vi "StopScan.vi"(0 "Close FP":bool, 1 "Motion Settings In":T5={"No Motion?"=FALSE, "Motion System"=enum."NI 735x", "Motion Bd ID"=1, "Motion Profile"="SMAC1", "# Axis"=1, "Reverse Z axis?"=TRUE, "SMAC Axis"=0, "scan pair"=enum."y-(x) scan", "RT fps"=6.0, "Steps per mm"=[1000, 1000, 1000, 1000], "Motor Parameters"={"velocity ct/s"=[10000.0, 10000.0, 10000.0, 50000.0], "accel ct/s^2"=[50000.0, 50000.0, 50000.0, 200000.0]}, "One Way Scan"=FALSE, "Reverse One Way Scan"=FALSE, "Global Position (mm)"=[], "Plane"=0, "Distance between\nscan lines (um)"=0.0, "Distance between\nscan planes (um)"=0.0, "number of scan planes"=1, "Total steps in line"=0, "Xtra plane\ndistance  (um)"=100, "Xtra planes "=1, "Add Axis"=FALSE, "overshoot cts"=200, "BKPT Shift"=0, "Scan Start Time (ms)"=0, "ESP VISA"="GPIB::1::INSTR", "3rd Axis"=1, "GL Ref Out"=refnum, "Galil Address"=""} {"3rd Axis" items=["x", "y", "z", "w"]; "Xtra planes" min=1; "Xtra plane\ndistance  (um)" min=0; "Distance between\nscan planes (um)" format="%.2f"; "Distance between\nscan lines (um)" format="%.2f"; "SMAC Axis" items=["None"=0, "Axis 1"=1, "Axis 2"=2, "Axis 3"=3, "Axis 4"=4, "Axis 5"=5, "Axis 6"=6, "Axis 7"=7, "Axis 8"=8, "Vector Space 1"=17, "Vector Space 2"=18, "Vector Space 3"=19, "Vector Space 4"=20]; "Motion Bd ID" min=1 max=32 step=1}, 2 "Ring":i32, 4 "Digitizer Settings":T1={"Digitizer delay (us) "=0.0, "rf points per line"=2048, "lines per plane"=128, "Samp Rate (Hz)"=100000000.0, "Additional dig delay (us)"=0.0, "Voltage Scale"=0.4, "Pre-Looks"=0, "Offset delay (us)"=0.0, "bits A/D"=8, "Avg Num"=1, "DigTimeOut"=5.0, "Rel Dig Delay"=0.0, "Dig Ch"=0, "LeCroyCluster"={"LeCroy Channels"=[TRUE, FALSE, FALSE, FALSE], "LC read pt offset"=0.0, "Sweep Avg"=FALSE}, "Main Digitizer"=enum."NI Digitizer", "Dig Config"=enum."Single channel", "Digitizer ID Cluster"={"Acqiris/Alazar/SP ID"=[], "NI Instr Handles"=[], "LeCroy VISA"="", "GaGe Handle"={"Handle"=0, "Sample size"=0, "Resolution"=0, "Offset"=0, "Channels"=0, "Boards"=0}, "ATS Ref"="ATS9350", "Acqiris Address"=["PCI::INSTR0"], "ADQRef"=refnum, "adq_cu_ptr"=refnum}, "Trigger Settings"={"Trig Source"=1, "Trig Coupling"=0, "Trig Slope"=0, "Level (mV)"=1500.0}, "Bulk Acq"=FALSE, "Bulk Start Indexes"=[], "Data Ref RF"=refnum, "NI ID/Channel"=[], "Total Dig CH"=1, "Xtra Ann Trig delay (us)"=10.0, "Fix Z Delay?"=FALSE, "One Way Transmission?"=FALSE, "Data Ref Log"=refnum} {"Trigger Settings"."Trig Slope" items=["Positive", "Negative"]; "Trigger Settings"."Level (mV)" format="%.2f"; "Trigger Settings"."Trig Coupling" items=["DC 1 MOhm", "AC 1 MOhm", "DC 50 Ohm", "AC 50 Ohm"]; "Trigger Settings"."Trig Source" items=["Chan 1", "External"]; "Rel Dig Delay" format="%.2f"; "DigTimeOut" format="%.2f"; "Avg Num" min=1; "Offset delay (us)" format="%.2f"; "Additional dig delay (us)" format="%.2f"; "Digitizer delay (us)" format="%.2f"}, 6 "Line Number":i32) -> (5 "Stop Now? Dup":bool)   [LabVIEW 2022 SP3]
uses:
  Motion Controllers/NI_controller/-NI_MotionRoutines/MotionParameters.ctl
  Motion Controllers/NI_controller/-NI_MotionRoutines/MotionSys.ctl
  Motion Controllers/-MotionRoutines/ScanAxis.ctl
  Motion Controllers/-MotionRoutines/3rdAxis.ctl
  Digitizers/-DigitizerRoutines/DigitizerSettings.ctl
  Digitizers/-DigitizerRoutines/Digitizer.ctl
  Digitizers/-DigitizerRoutines/DigConfig.ctl
  Digitizers/-DigitizerRoutines/DigitizerID.ctl
  C:/Windows/System32/ADQAPI_dotNet_helper.dll
panel:
  in  "Alert when done?":bool=TRUE
  out "Minutes Remaining":dbl format="%.1f"
  out "Progress":u8(slide) scale=0.0..100.0
  in  "Pause?":bool
  in  "Current Plane":i32
  in  "Stop Now?":bool
  # "Can pause or stop mid-scan"
  # "1-D and 2-D B scan settings"
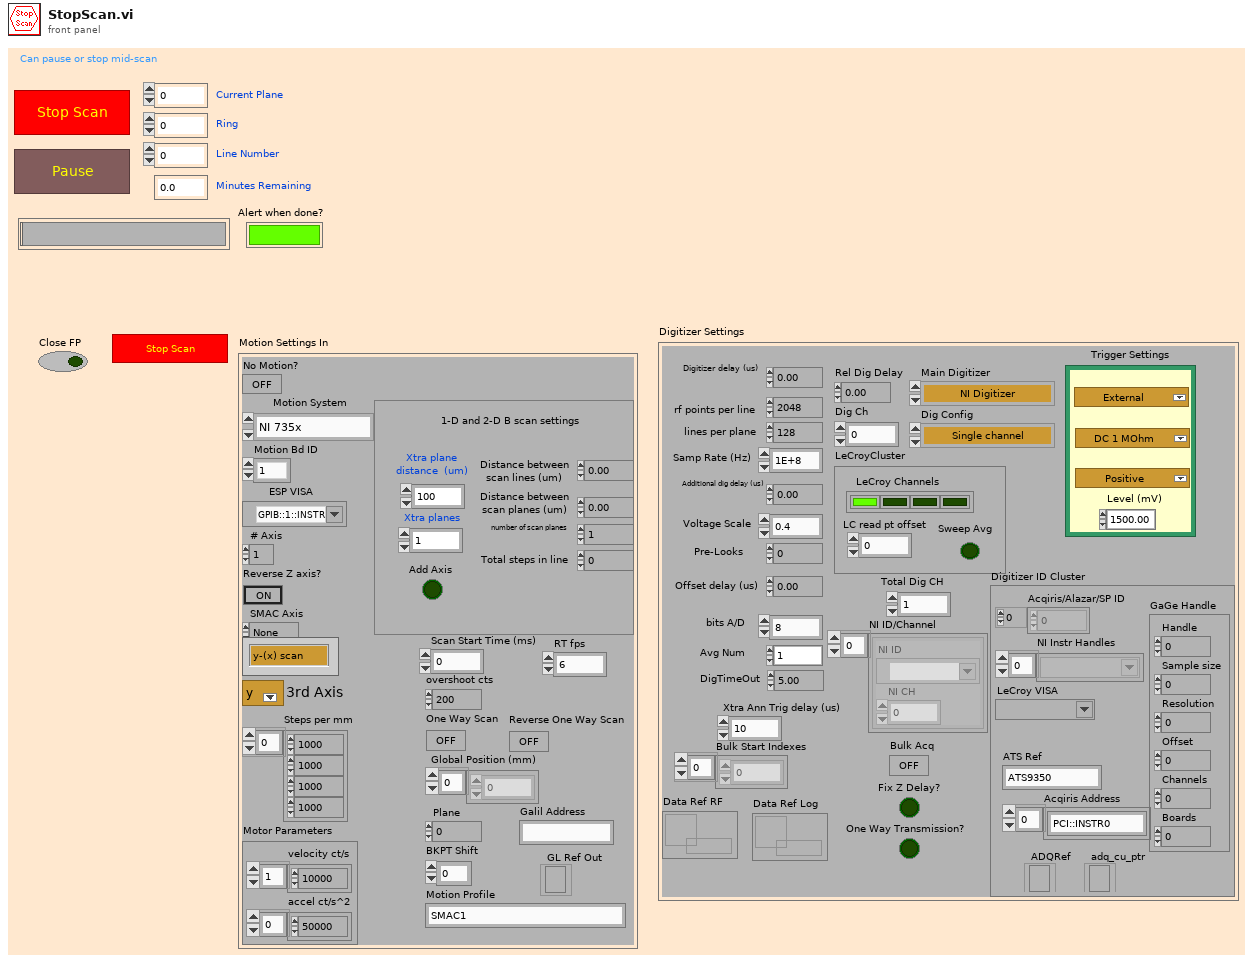
[diagram p1: front panel]
types:
  T1 = typedef "DigitizerSettings.ctl" = cluster{"Digitizer delay (us) ":dbl, "rf points per line":i32, "lines per plane":i32, "Samp Rate (Hz)":dbl, "Additional dig delay (us)":dbl, "Voltage Scale":dbl, "Pre-Looks":i32, "Offset delay (us)":dbl, "bits A/D":i8, "Avg Num":i32, "DigTimeOut":sgl, "Rel Dig Delay":sgl, "Dig Ch":i32, "LeCroyCluster":cluster{"LeCroy Channels":bool[], "LC read pt offset":dbl, "Sweep Avg":bool}, "Main Digitizer":T2, "Dig Config":T3, "Digitizer ID Cluster":T4, "Trigger Settings":cluster{"Trig Source":u16, "Trig Coupling":u16, "Trig Slope":u16, "Level (mV)":dbl}, "Bulk Acq":bool, "Bulk Start Indexes":i32[], "Data Ref RF":refnum<data-value>, "NI ID/Channel":cluster{"NI ID":refnum<k15>, "NI CH":i32}[], "Total Dig CH":i32, "Xtra Ann Trig delay (us)":dbl, "Fix Z Delay?":bool, "One Way Transmission?":bool, "Data Ref Log":refnum<data-value>}
  T2 = typedef "Digitizer.ctl" = enum16{"Acqiris Digitizer", "NI Digitizer", "LeCroy", "GaGe", "AlazarTech", "No Digitizer", "Teledyne"}
  T3 = typedef "DigConfig.ctl" = enum16{"Single channel", "2 Chans w/ 2 Acqiris", "2 Chans w/ 1 Acqiris", "5-CH Pulser New", "5-CH pulser w/ ann array", "5-pass style ann array", "Empty"}
  T4 = typedef "DigitizerID.ctl" = cluster{"Acqiris/Alazar/SP ID":u32[], "NI Instr Handles":refnum<k15>[], "LeCroy VISA":refnum<visa-resource-name>, "GaGe Handle":cluster{"Handle":u32, "Sample size":u32, "Resolution":i32, "Offset":i32, "Channels":u32, "Boards":u32}, "ATS Ref":string, "Acqiris Address":string[], "ADQRef":refnum<k24>, "adq_cu_ptr":refnum<k24>}
  T5 = typedef "MotionParameters.ctl" = cluster{"No Motion?":bool, "Motion System":T6, "Motion Bd ID":u8, "Motion Profile":string, "# Axis":i8, "Reverse Z axis?":bool, "SMAC Axis":u16, "scan pair":T7, "RT fps":sgl, "Steps per mm":i32[], "Motor Parameters":cluster{"velocity ct/s":dbl[], "accel ct/s^2":dbl[]}, "One Way Scan":bool, "Reverse One Way Scan":bool, "Global Position (mm)":dbl[], "Plane":i32, "Distance between\nscan lines (um)":sgl, "Distance between\nscan planes (um)":sgl, "number of scan planes":i32, "Total steps in line":i32, "Xtra plane\ndistance  (um)":i32, "Xtra planes ":i32, "Add Axis":bool, "overshoot cts":i32, "BKPT Shift":i32, "Scan Start Time (ms)":u32, "ESP VISA":refnum<visa-resource-name>, "3rd Axis":T8, "GL Ref Out":refnum<k7>, "Galil Address":string}
  T6 = typedef "MotionSys.ctl" = enum16{"MM3000", "NI 735x", "Newport ESP", "No Motion Card", "Galil"}
  T7 = typedef "ScanAxis.ctl" = enum16{"y-(x) scan", "x-(y) scan", "z-(x) scan", "z-(y) scan", "y-(z) scan", "x-(z) scan", "w-(x) scan", "w-(y) scan", "w-(z) scan", "x-(w) scan", "y-(w) scan", "z-(w) scan"}
  T8 = typedef "3rdAxis.ctl" = u16
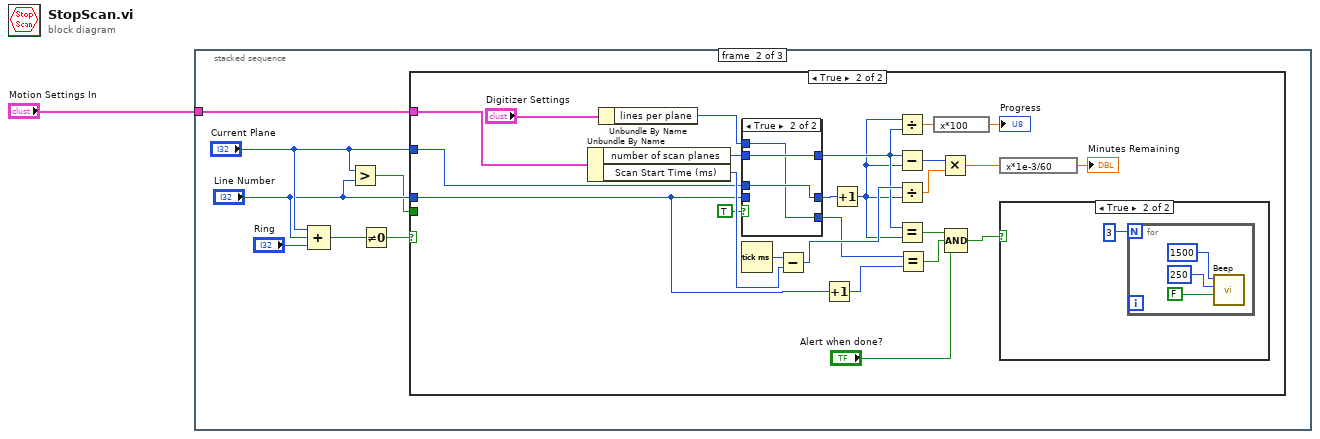
[diagram p0: block diagram]
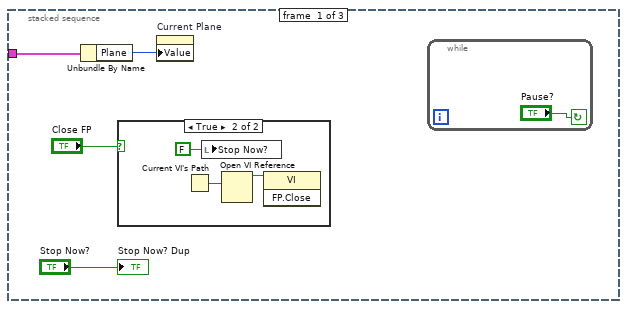
[diagram p2: hidden frame]
diagram:
  n1 = stacked-sequence {
    tunnel: "Motion Settings In" -> [w2 w10 _]
    frame #0 {
      n2 = Unbundle By Name(w2) -> ("Plane"=w3:i32)
      n3 = case shown="True" "Close FP" {
        frame False {
        }
        frame True {
          n4 = Current VI's Path() -> (path=w9:path)
          n5 = local write "Stop Now?"(FALSE) -> ()
          n6 = Open VI Reference(vi path=w9) -> (vi reference=w8:refnum<vi>)  [unwired: 2 in, 4 out]
          n7 = invoke class="VI" method="FP.Close"(reference=w8) -> ()  [unwired: 2 in, 3 out]
        }
      }
      n8 = property on="Current Plane" class="DigNum (strict)"("Value"=w3) -> ()  [unwired: 2 in, 2 out]
      n9 = while {
        stop <- "Pause?" continue-if-true
      }
      "Stop Now? Dup" <- "Stop Now?"
    }
    frame #1 {
      n10 = Compound Arithmetic op=ADD("Current Plane", "Line Number", "Ring") -> (w16:i32)
      n11 = Greater?(x="Current Plane", y="Line Number") -> (0:w11:bool)
      n12 = Not Equal To 0?(x=w16) -> (x != 0?=w15:bool)
      n13 = case shown="True" w15 {
        tunnel: "Current Plane" -> [_ w28]
        tunnel: w11 -> [_ _]
        tunnel: "Line Number" -> [_ w18]
        tunnel: w10 -> [_ w24]
        frame False {
        }
        frame True {
          n14 = Unbundle By Name(w24) -> ("number of scan planes"=w26:i32, "Scan Start Time (ms)"=w33:u32)
          n15 = Unbundle By Name("Digitizer Settings") -> ("lines per plane"=w25:i32)
          n16 = case shown="True" TRUE {
            tunnel: [w43 w46] -> w29
            tunnel: w28 -> [_ w46]
            tunnel: w18 -> [w43 _]
            tunnel: [w42 w45] -> w27
            tunnel: w26 -> [_ w45]
            tunnel: w25 -> [w42 w44]
            tunnel: [w42 w44] -> w22
            frame False {
            }
            frame True {
            }
          }
          n17 = Tick Count (ms)() -> (millisecond timer value=w41:u32)
          n18 = Subtract(x=w41, y=w33) -> (x-y=w34:u32)
          n19 = Increment(x=w18) -> (x+1=w17:i32)
          n20 = Increment(x=w29) -> (x+1=w21:i32)
          n21 = Divide(x=w21, y=w27) -> (x/y=w40:dbl)
          n22 = Subtract(x=w27, y=w21) -> (x-y=w39:i32)
          n23 = Divide(x=w34, y=w21) -> (x/y=w38:dbl)
          n24 = Equal?(x=w27, y=w21) -> (x = y?=w31:bool)
          n25 = Equal?(x=w22, y=w17) -> (x = y?=w20:bool)
          n26 = expression code="x*100"(w40) -> (→"Progress":dbl)
          n27 = Multiply(x=w39, y=w38) -> (x*y=w37:dbl)
          n28 = Compound Arithmetic op=AND(w31, w20, "Alert when done?") -> (w32:bool)
          n29 = expression code="x*1e-3/60"(w37) -> (→"Minutes Remaining":dbl)
          n30 = case shown="True" w32 {
            frame False {
            }
            frame True {
              n31 = for {
                N: 3 -> [_]
                n32 = call <vilib>:"Beep.vi"("use system alert? (T)"=FALSE, "duration (msec)"=u32 250, "frequency (Hz)"=u32 1500) -> ()  [unwired: 9 in]
              }
            }
          }
        }
      }
    }
    frame #2 {
    }
  }
